vi "Apply Selected Labels to Control.vi"(8 "error in (no error)":errorcluster, 10 "Alternate Text Select (0)":i32, 11 "Combo Box in":refnum<class "Combo Box.lvclass">) -> (0 "error out":errorcluster, 3 "Combo Box out":refnum<class "Combo Box.lvclass">)   [LabVIEW 2017, in "Localization.lvlib" / "Combo Box.lvclass"]
doc: "Use the information in the class to apply the selected alternate text from the Additional Labels to the control.\n\nChoose Movement Consulting, LLC"
uses:
  Combo Box.lvclass
  C:/Apps/CMC/OpenSource/Localization/Control Info/Control Info.lvclass
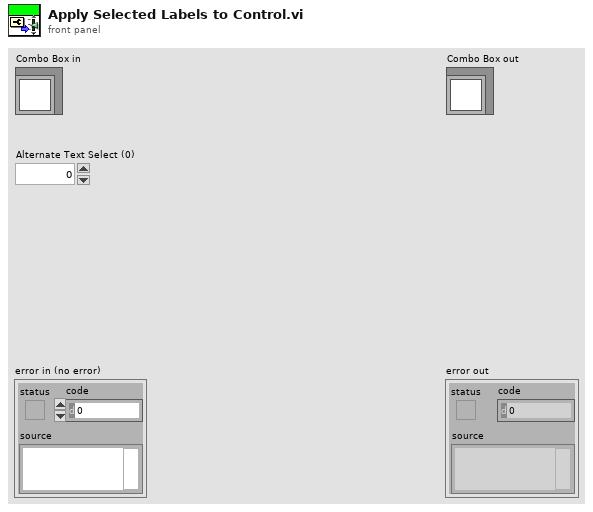
[diagram p1: front panel]
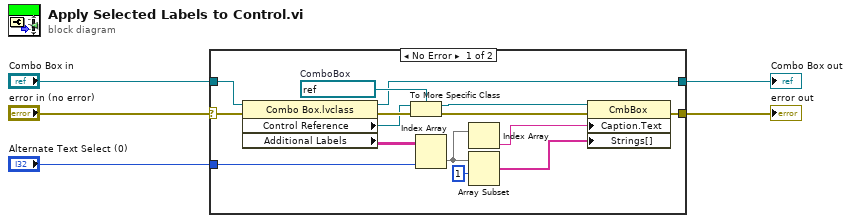
[diagram p0: block diagram]
diagram:
  n1 = case shown="No Error" "error in (no error)" {
    selector: "error in (no error)" -> [w15 w22]
    tunnel: "Combo Box in" -> [w14 w21]
    tunnel: [w8 w22] -> w1
    tunnel: [w7 w21] -> w2
    tunnel: "Alternate Text Select (0)" -> [w12 _]
    frame No Error {
      w20 = refnum<vi> refnum  # ComboBox
      n2 = property class="Combo Box.lvclass"(reference=w14, error in=w15) -> (reference out=w7:refnum<class "Combo Box.lvclass">, error out=w17:errorcluster, "Control Reference"=w16:refnum<vi>, "Additional Labels"=w13:string[][])
      n3 = To More Specific Class(target class=w20, reference=w16, error in=w17) -> (specific class reference=w19:refnum<vi>, error out=w18:errorcluster)
      n4 = Index Array(array=w13, index (col)=w12) -> (element=w10:string[])  [unwired: 1 in]
      n5 = Index Array(array=w10) -> (element=w11:string)  [unwired: 1 in]
      n6 = Array Subset(array=w10, index=1) -> (w6:string[])  [unwired: 1 in]
      n7 = property class="CmbBox"(reference=w19, error in=w18, "Caption.Text"=w11, "Strings[]"=w6) -> (error out=w8:errorcluster)  [unwired: 1 out]
    }
    frame Error {
    }
  }
  "error out" <- w1
  "Combo Box out" <- w2
